vi "Init Condition.vi"(5 "Sequencing":refnum<class "MessageQ.lvclass">, 6 "Variables":refnum<class "Variables.lvclass">, 7 "VolatusAPI":refnum<class "VolatusAPI.lvclass">, 8 "error in (no error)":refnum<class "MultiErrors.lvclass">, 10 "Condition Config":refnum<class "Condition Config.lvclass">, 11 "SeqLoaded Condition in":refnum<class "SeqLoaded Condition.lvclass">) -> (0 "error out":refnum<class "MultiErrors.lvclass">, 3 "SeqLoaded Condition out":refnum<class "SeqLoaded Condition.lvclass">)   [LabVIEW 2020, in "VolatusSeq.lvlib" / "SeqLoaded Condition.lvclass"]
uses:
  SeqLoaded Condition.lvclass
  VolatusErrorUtilities/MultiErrors/MultiErrors.lvclass
  Volatus/VolatusAPI/VolatusAPI.lvclass
  VolatusSeqConfig/Condition Config/Condition Config.lvclass
  Volatus/MessageQ/MessageQ.lvclass
  VolatusSeqConfig/SeqLoaded Condition Config/SeqLoaded Condition Config.lvclass
  SeqLoaded Condition.lvclass/SeqLoaded Condition.ctl
  Variables/Variables.lvclass
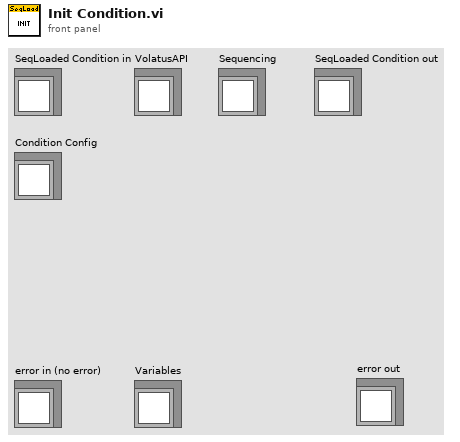
[diagram p1: front panel]
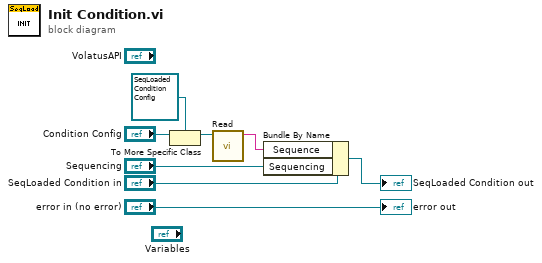
[diagram p0: block diagram]
diagram:
  n1 = To More Specific Class(target class=refnum<class "SeqLoaded Condition Config.lvclass"> refnum ("VolatusSeqConfig.lvlib:SeqLoaded Condition Config.lvclass"), reference="Condition Config") -> (specific class reference=w5:refnum<class "SeqLoaded Condition Config.lvclass">)  [unwired: 1 in, 1 out]
  n2 = call "Read.vi"("SeqLoaded Condition Config in"=w5) -> ("Sequence"=w2:string)  [unwired: 10 in]
  n3 = Bundle By Name(cluster="SeqLoaded Condition in", "Sequence"=w2, "Sequencing"="Sequencing") -> (→"SeqLoaded Condition out":refnum<class "SeqLoaded Condition.lvclass">)
  "error out" <- "error in (no error)"
